vi "Sub Panel Call VI.vi"(8 "error in (no error)":errorcluster, 10 "name or relative path":string, 11 "base path":path) -> (0 "error out":errorcluster, 3 "VI Refnum":refnum<vi>)   [LabVIEW 2021]
doc: "SubPanel call a vi.\n2015-03-03 12:55:53\n蒋松\njiangsong@outlook.com"
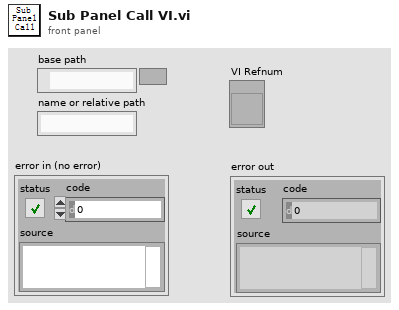
[diagram p1: front panel]
types:
  T1 = enum32{"Invalid", "Standard", "Closed", "Hidden", "Minimized", "Maximized"}
  T2 = enum32{"Bad", "Idle", "Run top level", "Running"}
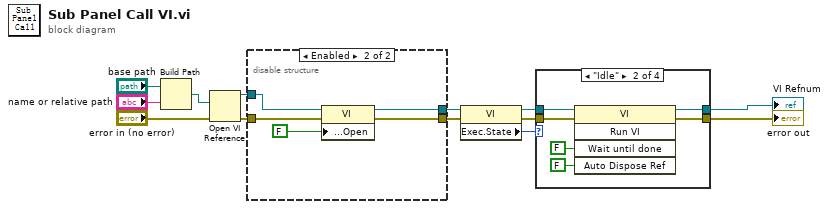
[diagram p0: block diagram]
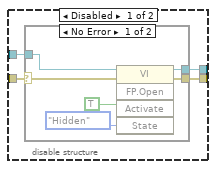
[diagram p2: hidden frame]
diagram:
  n1 = Build Path(base path="base path", name or relative path="name or relative path") -> (appended path=w13:path)
  n2 = Open VI Reference(vi path=w13, error in (no error)="error in (no error)") -> (vi reference=w11:refnum<vi>, error out=w12:errorcluster)  [unwired: 4 in]
  n3 = disable-structure shown="Enabled" {
    disable-tunnel: w12 -> [w17 w27]
    disable-tunnel: w11 -> [w16 w29]
    disable-tunnel: [w15 w26] -> w10
    disable-tunnel: [w14 w28] -> w6
    frame Disabled {
      n4 = case shown="No Error" w17 {
        selector: w17 -> [w18 w24]
        tunnel: [w21 w24] -> w15
        tunnel: w16 -> [w20 w25]
        tunnel: [w19 w25] -> w14
        frame No Error {
          n5 = invoke class="VI" method="FP.Open"(reference=w20, error in=w18, "Activate"=TRUE, "State"=T1."Hidden") -> (reference out=w19:refnum<vi>, error out=w21:errorcluster)  [unwired: 1 in, 3 out]
        }
        frame Error {
        }
      }
    }
    frame Enabled {
      n6 = property class="VI"(reference=w29, error in=w27, "Front Panel Window:Open"=FALSE) -> (reference out=w28:refnum<vi>, error out=w26:errorcluster)
    }
  }
  n7 = property class="VI"(reference=w6, error in=w10) -> (reference out=w8:refnum<vi>, error out=w7:errorcluster, "Exec.State"=w9:T2)
  n8 = case shown="\"Idle\"" w9 {
    tunnel: w8 -> [w32 w36 w40 w42]
    tunnel: w7 -> [w31 w35 w39 w41]
    tunnel: [w32 w34 w40 w42] -> w1
    tunnel: [w31 w33 w39 w41] -> w2
    frame "Bad", Default {
    }
    frame "Idle" {
      n9 = invoke class="VI" method="Run VI"(reference=w36, error in=w35, "Wait until done"=FALSE ("Wait Until Done"), "Auto Dispose Ref"=FALSE ("Auto Dispose Reference")) -> (reference out=w34:refnum<vi>, error out=w33:errorcluster)  [unwired: 1 in, 3 out]
    }
    frame "Run top level" {
    }
    frame "Running" {
    }
  }
  "error out" <- w2
  "VI Refnum" <- w1
